vi "Remove Value.vi"(8 "error in (no error)":errorcluster, 10 "key":string, 11 "JSON Object in":refnum<class "JSON Value.lvclass">) -> (0 "error out":errorcluster, 2 "found":bool, 3 "JSON Object out":refnum<class "JSON Value.lvclass">)   [LabVIEW 2016, in "JSON Value.lvclass"]
doc: "Remove the given parameter from the specified JSON Object"
uses:
  JSON Helper/JSON Value.lvclass
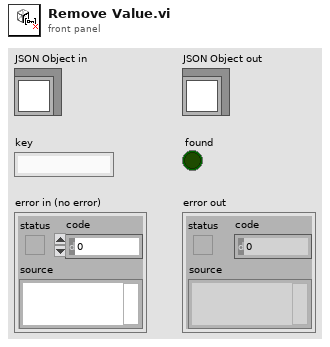
[diagram p1: front panel]
types:
  T1 = typedef "JSON Value.lvclass/JSON Types.ctl" = enum16{"String", "Numeric", "Boolean", "NULL", "Object", "Array"}
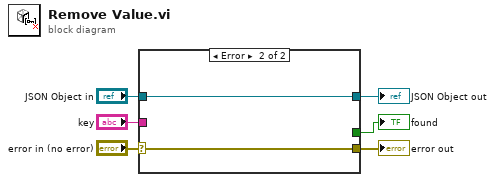
[diagram p0: block diagram]
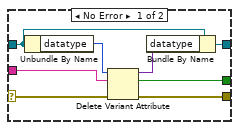
[diagram p2: hidden frame]
diagram:
  n1 = case shown="Error" "error in (no error)" {
    selector: "error in (no error)" -> [w13 w16]
    tunnel: [w11 w16] -> w5
    tunnel: "JSON Object in" -> [w9 w15]
    tunnel: "key" -> [w14 _]
    tunnel: [w10 _] -> w2
    tunnel: [w7 w15] -> w1
    frame No Error {
      n2 = Unbundle By Name(w9) -> ("datatype"=w12:T1)
      n3 = Delete Variant Attribute(4:w13, 6:w14, 7:w12) -> (0:w11:errorcluster, 2:w10:bool, 3:w8:variant)
      n4 = Bundle By Name(cluster=w9, "datatype"=w8) -> (w7:refnum<class "JSON Value.lvclass">)
    }
    frame Error {
    }
  }
  "error out" <- w5
  "found" <- w2
  "JSON Object out" <- w1
